vi "DS1820TEMP.vi"() -> ()   [LabVIEW 2017]
uses:
  <vilib>/LabVIEW Interface for Arduino/Type Defs/Pin Mode.ctl
  <vilib>/Instr/_visa.llb/VISA Configure Serial Port (Instr).vi
  <vilib>/LabVIEW Interface for Arduino/LabVIEW Interface for Arduino.lvlib
panel:
  in  "stop":bool
  in  "Lim_inf":dbl
  in  "Lim_sup":dbl
  out "WAVE TEMP":i32(graph)
  out "TEMP GAUGE":dbl(slide) scale=0.0..100.0
  out "TEMP":string
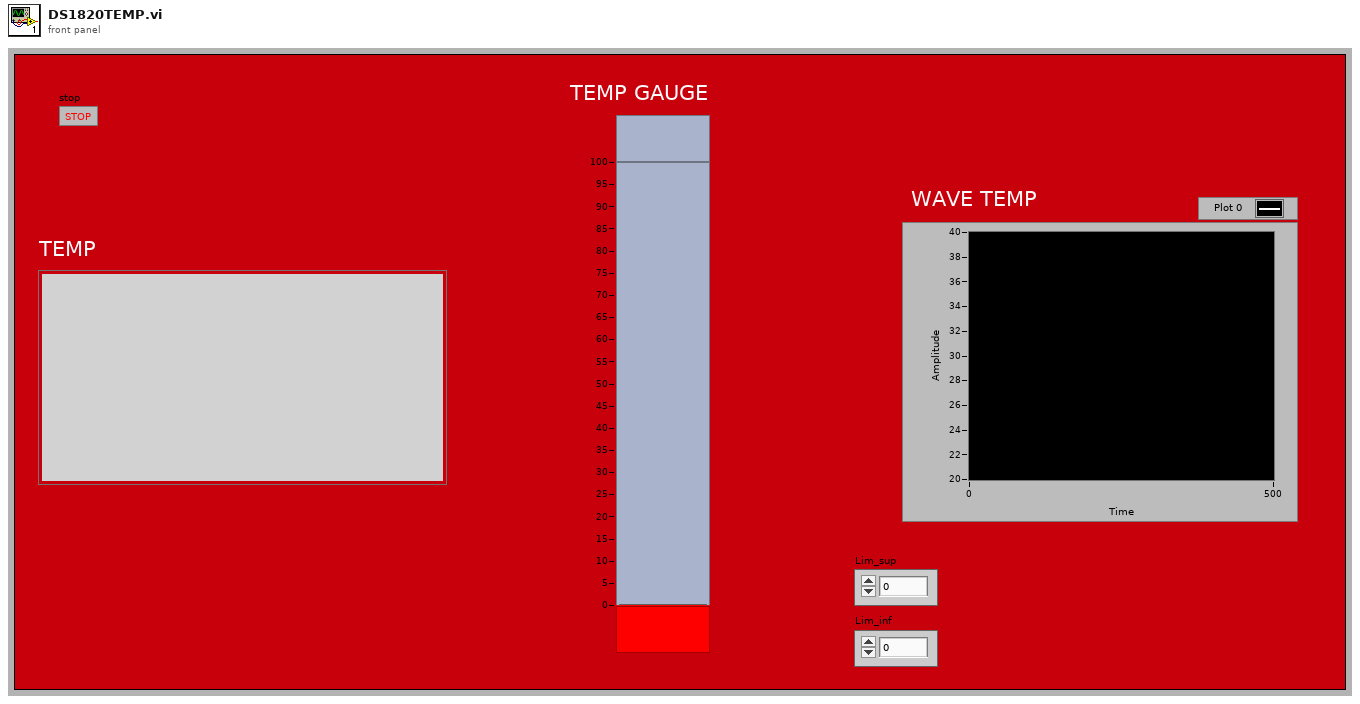
[diagram p1: front panel]
types:
  T1 = typedef "LabVIEW Interface for Arduino.lvlib/Arduino Resource.ctl" = cluster{"VISA resource":refnum<visa-resource-name>, "Board Type":T2, "Connection Type":enum8{"USB / Serial"}, "Bytes Per Packet (15)":u8}
  T2 = typedef "LabVIEW Interface for Arduino.lvlib/Board Type.ctl" = enum16{"Uno", "Dimuelanove w/Atmega 328", "Mega 2560"}
  T3 = typedef "LabVIEW Interface for Arduino.lvlib/Pin Mode.ctl" = enum8{"Input", "Output"}
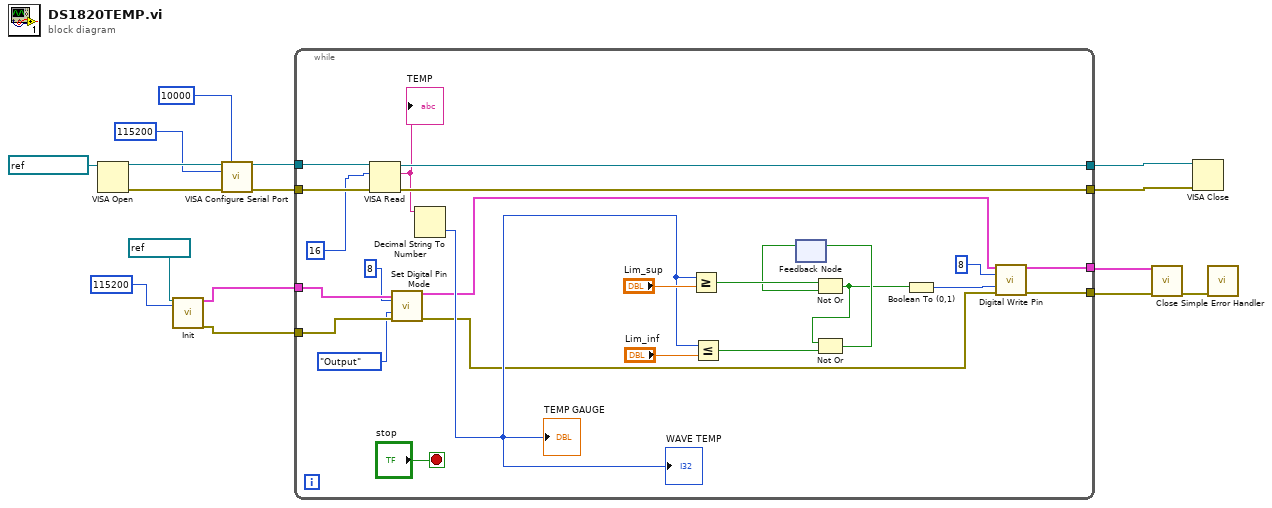
[diagram p0: block diagram]
diagram:
  n1 = VISA Open(VISA resource name=refnum<visa-resource-name> "COM3") -> (VISA resource name=w12:refnum<visa-resource-name>, error out=w11:errorcluster)  [unwired: 4 in]
  n2 = call <vilib>:"Init.vi"("VISA resource"=refnum<visa-resource-name> "COM3", "Baud Rate (115200)"=u32 115200) -> ("Arduino Resource"=w2:T1, "error out"=w1:errorcluster)  [unwired: 16 in]
  n3 = call-poly "VISA Configure Serial Port"("VISA resource name"=w12, "timeout (10sec)"=u32 10000, "baud rate (9600)"=u32 115200, "error in (no error)"=w11) -> ("VISA resource name out"=w14:refnum<visa-resource-name>, "error out"=w13:errorcluster)  [unwired: 10 in]
  n4 = while {
    tunnel: [w41] -> w16
    tunnel: [w40] -> w15
    tunnel: w14 -> [w39]
    tunnel: w13 -> [w38]
    tunnel: [w25] -> w9
    tunnel: [w24] -> w8
    tunnel: w2 -> [w22]
    tunnel: w1 -> [w21]
    stop <- "stop" stop-if-true
    n5 = VISA Read(VISA resource name=w39, byte count=u32 16, error in (no error)=w38) -> (VISA resource name out=w41:refnum<visa-resource-name>, read buffer=w37:string, error out=w40:errorcluster)  [unwired: 1 out]
    "TEMP" <- w37
    n6 = call <vilib>:"Set Digital Pin Mode.vi"("Arduino Resource"=w22, "Digital I/O Pin"=u8 8, "Pin Mode (Input)"=Pin_Mode."Output", "error in"=w21) -> ("Arduino Resource"=w20:T1, "error out"=w19:errorcluster)  [unwired: 10 in]
    n7 = Decimal String To Number(string=w37) -> (number=w29:i32)  [unwired: 2 in, 1 out]
    "TEMP GAUGE" <- w29
    "WAVE TEMP" <- w29
    n8 = Greater Or Equal?(x=w29, y="Lim_sup") -> (x >= y?=w34:bool)
    n9 = Less Or Equal?(x=w29, y="Lim_inf") -> (x <= y?=w35:bool)
    n10 = feedback #1() -> (w33:bool)  [unwired: 1 in]
    n11 = Not Or(1:w33, 2:w34) -> (0:w27:bool)
    n12 = Not Or(1:w35, 2:w27) -> (0:w32:bool)
    n13 = feedback-in #1(w32) -> ()
    n14 = Boolean To (0,1)(Boolean=w27) -> (0, 1=w26:i16)
    n15 = call <vilib>:"Digital Write Pin.vi"("Arduino Resource"=w20, "Digital I/O Pin (0)"=u32 8 ("byte count"), "Value (0)"=w26, "error in"=w19) -> ("Arduino Resource"=w25:T1, "error out"=w24:errorcluster)  [unwired: 10 in]
  }
  n16 = call <vilib>:"Close.vi"("Arduino Resource"=w9, "error in"=w8) -> ("error out"=w7:errorcluster)  [unwired: 13 in]
  n17 = VISA Close(VISA resource name=w16, error in (no error)=w15) -> ()  [unwired: 1 out]
  n18 = call <vilib>:"Simple Error Handler.vi"("error in (no error)"=w7) -> ()  [unwired: 4 in, 5 out]
